vi "control.vi"(5 "control":T9={"time (global)"=0.0, "MPV"=0, "manual control"={"sequence manual"=enum."WAIT", "sequence manual ?"=FALSE}}, 6 "sequenzen":T4, 7 "command parameter":T6={"CO2 ref"=392.0, "CO2 span"=372.0, "H2O ref"=0.0, "H2O span"=0.0, "Zi"=0.0, "Zt"=1.2, "Zm"=0.0, "S"=0.0, "Temp [C]"=50.0, "Pressure [hPa]"=135.0, "Licor-Sources"=["CO2A W", "CO2B W", "H2OA W", "H2OB W", "T C", "T V", "P kPa", "P V", "RH %", "CO2A um/m", "CO2B um/m", "H2OA mm/m", "H2OB mm/m"], "Licor-Pump"="Off", "Zeitstempel"=timestamp(0 s since 1904-01-01)} {"Pressure [hPa]" format="%_5g"; "Temp [C]" format="%.2f"; "CO2 ref" format="%.2f"; "CO2 span" format="%.2g"; "H2O ref" format="%.2g"; "H2O span" format="%.2g"; "Zt" format="%#_4g"}, 8 "Licor-output":T5[](array[typedef]) {"time (global)" format="%<%H:%M:%S\n%d/%m/%Y>T"}, 9 "sequence in":T2={"sequence"=enum."WAIT", "Zeitpunkt next"=0.0, "delta t"=0.0} {"Zeitpunkt next" format="%<%H:%M:%S%3u>T"}, 11 "command queue in":cluster{"Zeit [s]":i32, "Befehl":string}[](array[cluster])) -> (0 "Licor command":string, 1 "sequence out":T2={"sequence"=enum."WAIT", "Zeitpunkt next"=0.0, "delta t"=0.0} {"Zeitpunkt next" format="%<%H:%M:%S%3u>T"}, 3 "command queue out":cluster{"Zeit [s]":i32, "Befehl":string}[](array[cluster]), 4 "data":T5[](array[typedef]) {"time (global)" format="%<%H:%M:%S\n%d/%m/%Y>T"})   [LabVIEW 2017, in "Licor-Steuerung.lvlib"]
uses:
  Licor-Steuerung.lvlib
  Licor-Sequences.ctl
  Licor-Parameter.ctl
  LicorLI7000/conventions/Licor-Source.ctl
  Licor-Pump.ctl
  LicorLI7000/conventions/output line.ctl
  Licor-Commands.ctl
  LicorLI7000/LicorLI7000.lvlib
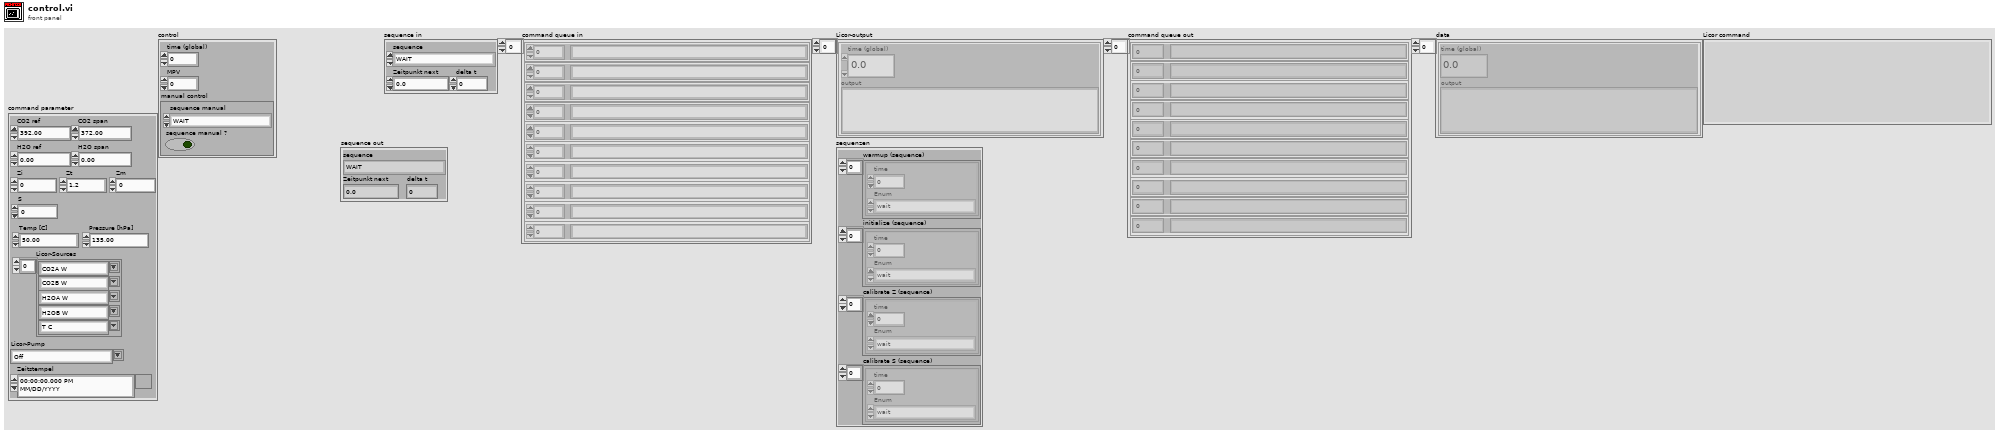
[diagram p1: front panel]
types:
  T1 = typedef "Licor-Steuerung.lvlib/Licor-Sequences.ctl" = enum16{"test", "WAIT", "warmup", "initialize", "calibrate Z", "calibrate S"}
  T2 = cluster{"sequence":T1, "Zeitpunkt next":dbl, "delta t":dbl}
  T3 = typedef "Licor-Steuerung.lvlib/Licor-Commands.ctl" = enum16{"wait", "initialize", "resetCO2", "resetH2O", "getReference", "setReference", "calibration-Z-CO2", "calibration-Z-H2O", "calibration-S-CO2", "calibration-S-H2O", "getCalibrationParameter", "setZeroParameter", "setLicorTime", "getLicorTime", "setPumpFlowrate", "setPumpSlow", "setPumpMedium", "setPumpFast", "getInfo"}
  T4 = cluster{"warmup (sequence)":cluster{"time":i32, "Enum":T3}[], "initialize (sequence)":cluster{"time":i32, "Enum":T3}[], "calibrate Z (sequence)":cluster{"time":i32, "Enum":T3}[], "calibrate S (sequence)":cluster{"time":i32, "Enum":T3}[]}
  T5 = typedef "LicorLI7000.lvlib/output line.ctl" = cluster{"time (global)":dbl, "output":string}
  T6 = typedef "Licor-Steuerung.lvlib/Licor-Parameter.ctl" = cluster{"CO2 ref":dbl, "CO2 span":dbl, "H2O ref":dbl, "H2O span":dbl, "Zi":dbl, "Zt":dbl, "Zm":dbl, "S":dbl, "Temp [C]":dbl, "Pressure [hPa]":dbl, "Licor-Sources":T7[], "Licor-Pump":T8, "Zeitstempel":timestamp}
  T7 = typedef "LicorLI7000.lvlib/Licor-Source.ctl" = string
  T8 = typedef "Licor-Steuerung.lvlib/Licor-Pump.ctl" = string
  T9 = cluster{"time (global)":dbl, "MPV":i32, "manual control":cluster{"sequence manual":T1, "sequence manual ?":bool}}
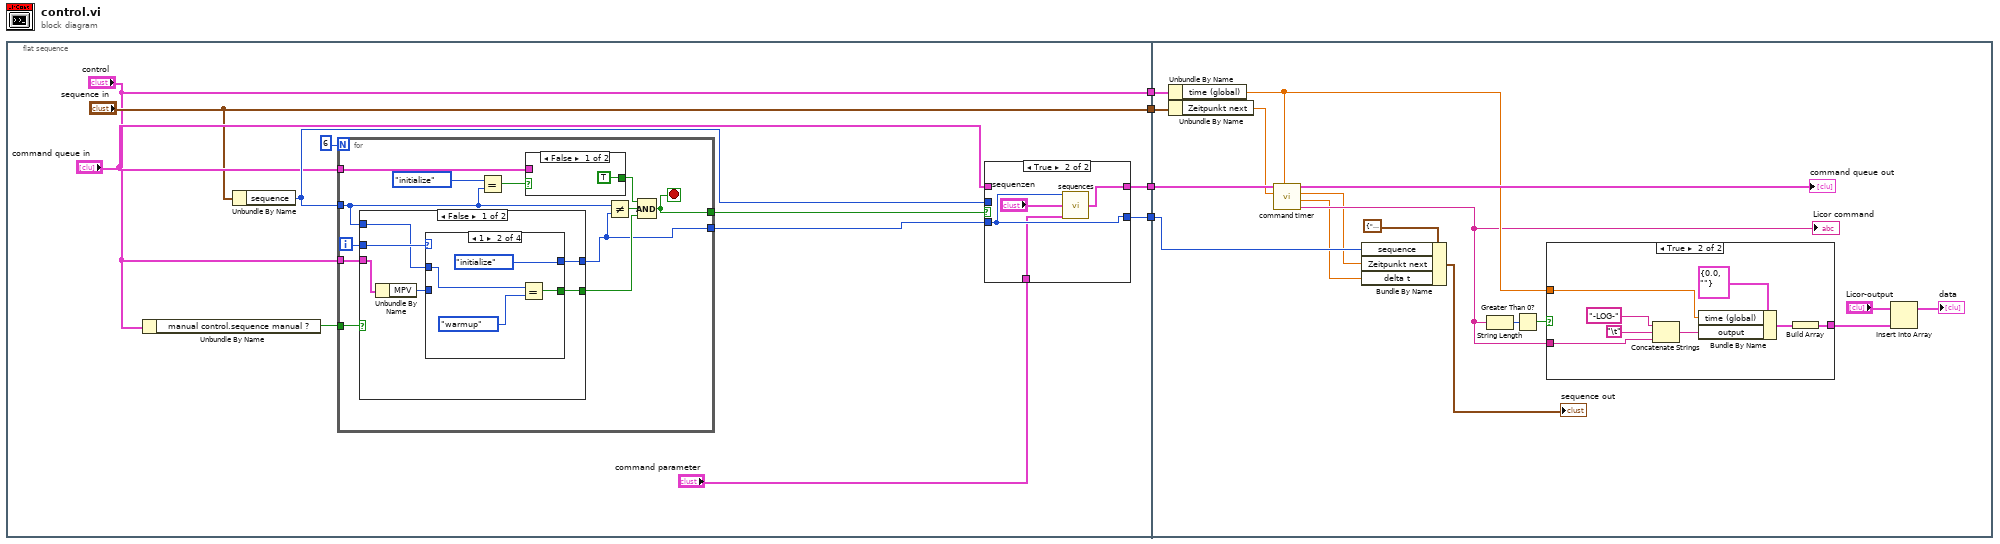
[diagram p0: block diagram]
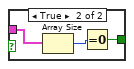
[diagram p3: hidden frame]
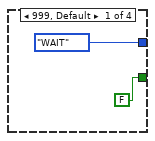
[diagram p4: hidden frame]
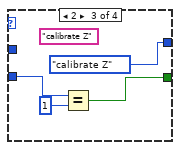
[diagram p5: hidden frame]
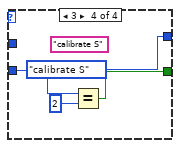
[diagram p6: hidden frame]
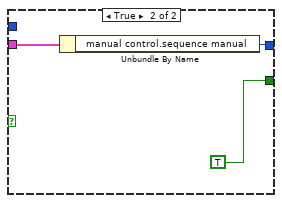
[diagram p7: hidden frame]
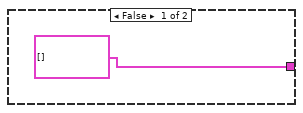
[diagram p8: hidden frame]
diagram:
  n1 = flat-sequence {
    tunnel: [w13] -> w4
    tunnel: [w11] -> w3
    tunnel: ["control"] -> w2
    tunnel: ["sequence in"] -> w1
    tunnel: w1 -> [w73]
    tunnel: w2 -> [w74]
    tunnel: w3 -> [w64]
    tunnel: w4 -> [w76]
    frame #0 {
      n2 = Unbundle By Name("control") -> ("manual control.sequence manual ?"=w14:bool)
      n3 = Unbundle By Name("sequence in") -> ("sequence"=w12:T1)
      n4 = for {
        N: 6 -> [_]
        tunnel: w12 -> [w22]
        tunnel: w14 -> [w30]
        tunnel: "control" -> [w29]
        tunnel: [w24] -> w10
        tunnel: [w28] -> w9
        tunnel: "command queue in" -> [w27]
        i -> [w33]
        stop <- w28 stop-if-true
        n5 = case shown="False" w30 {
          tunnel: w33 -> [w43 _]
          tunnel: [w42 w59] -> w24
          tunnel: [w41 TRUE] -> w31
          tunnel: w22 -> [w40 _]
          tunnel: w29 -> [w38 w60]
          frame False {
            n6 = Unbundle By Name(w38) -> ("MPV"=w39:i32)
            n7 = case shown="1" w43 {
              tunnel: w39 -> [_ _ w53 w56]
              tunnel: [FALSE w48 w51 w55] -> w41
              tunnel: [Licor-Sequences."WAIT" Licor-Sequences."initialize" Licor-Sequences."calibrate Z" Licor-Sequences."calibrate S"] -> w42
              tunnel: w40 -> [_ w49 _ _]
              frame 999, Default {
              }
              frame 1 {
                n8 = Equal?(x=w49, y=Licor-Sequences."warmup") -> (x = y?=w48:bool)
              }
              frame 2 {
                (unwired) "calibrate Z" ("sequence")
                n9 = Equal?(x=w53, y=1) -> (x = y?=w51:bool)
              }
              frame 3 {
                (unwired) "calibrate S" ("sequence")
                n10 = Equal?(x=w56, y=2) -> (x = y?=w55:bool)
              }
            }
          }
          frame True {
            n11 = Unbundle By Name(w60) -> ("manual control.sequence manual"=w59:T1)
          }
        }
        n12 = Equal?(x=Licor-Sequences."initialize", y=w22) -> (x = y?=w26:bool)
        n13 = case shown="False" w26 {
          tunnel: w27 -> [_ w36]
          tunnel: [TRUE w35] -> w25
          frame False {
          }
          frame True {
            n14 = Array Size(array=w36) -> (size(s)=w37:i32)
            n15 = Equal To 0?(x=w37) -> (x = 0?=w35:bool)
          }
        }
        n16 = Not Equal?(x=w22, y=w24) -> (x != y?=w32:bool)
        n17 = Compound Arithmetic op=AND(w25, w32, w31) -> (w28:bool)
      }
      n18 = case shown="True" w9 {
        tunnel: "command queue in" -> [w17 _]
        tunnel: [w17 w21] -> w13
        tunnel: w12 -> [w16 _]
        tunnel: [w16 w20] -> w11
        tunnel: w10 -> [_ w20]
        tunnel: "command parameter" -> [_ w19]
        frame False {
        }
        frame True {
          n19 = call "sequences.vi"("sequence"=w20, "sequenzen"="sequenzen", "command parameter"=w19) -> ("sequence out"=w21:cluster{"time":i32, "command":string}[])  [unwired: 12 in]
        }
      }
    }
    frame #1 {
      n20 = Unbundle By Name(w74) -> ("time (global)"=w72:dbl)
      n21 = Unbundle By Name(w73) -> ("Zeitpunkt next"=w69:dbl)
      n22 = call "command timer.vi"("time (global)"=w72, "time (next command)"=w69, "command queue in"=w76) -> ("Licor command"=w68:string, "x-y"=w61:dbl, "time (next command)"=w62:dbl, "command queue out"=→"command queue out":cluster{"Zeit [s]":i32, "Befehl":string}[])  [unwired: 5 in]
      "Licor command" <- w68
      n23 = Bundle By Name(cluster=T2 {"sequence"=enum."WAIT", "Zeitpunkt next"=0.0, "delta t"=0.0} ("sequence in"), "sequence"=w64, "Zeitpunkt next"=w62, "delta t"=w61) -> (→"sequence out":T2)
      n24 = String Length(string=w68) -> (length=w71:i32)
      n25 = Greater Than 0?(x=w71) -> (x > 0?=w70:bool)
      n26 = case shown="True" w70 {
        tunnel: w72 -> [_ w85]
        tunnel: w68 -> [_ w81]
        tunnel: [T5[] [] ("Licor-output 3") w83] -> w77
        frame False {
        }
        frame True {
          n27 = Concatenate Strings("-LOG-", "\t", w81) -> (w79:string)
          n28 = Bundle By Name(cluster=T5 {"time (global)"=0.0, "output"=""} ("output line"), "time (global)"=w85, "output"=w79) -> (w84:T5)
          n29 = Build Array(w84) -> (w83:T5[])
        }
      }
      n30 = Insert Into Array(array="Licor-output", new element=w77) -> (→"data":T5[])  [unwired: 1 in]
    }
  }
